vi "ZeroCalN1911a.vi"(2 "error in (no error)":errorcluster) -> (0 "error out":errorcluster)   [LabVIEW 2009]
doc: "Calibrates N1911A for average power measurements and disable automatic cal selection. Zeroing and calibration consume approximately 12 seconds.\nRecommend very low power into the N1921A sensor."
panel:
  in  "SCPI zero and cal commands":string="*cls\nCAL:ALL\nCAL:AUTO OFF\n\n"
  # "Calibrates N1911A for average power measurements and disable automatic cal selection. Zeroing and calibration consume approximately 12 seconds.\nRecommend very low power into the N1921A sensor."
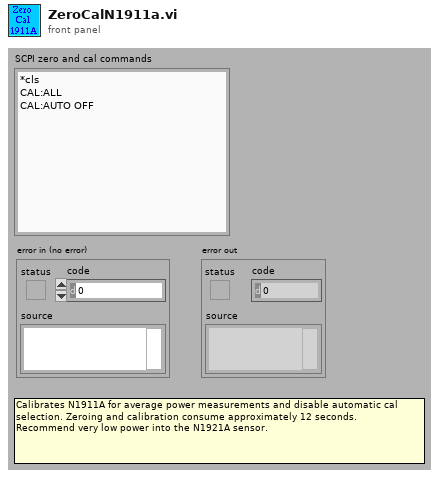
[diagram p1: front panel]
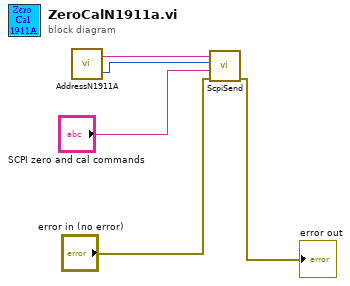
[diagram p0: block diagram]
diagram:
  n1 = call "AddressN1911A.vi"() -> ("Port"=w2:i32, "IP address"=w3:string)  [unwired: 2 in]
  n2 = call "ScpiSend.vi"("error in (no error)"="error in (no error)", "Command"="SCPI zero and cal commands", "TCP port"=w2, "IP Address"=w3) -> ("error out"=→"error out":errorcluster)  [unwired: 7 in]
